vi "hidSPD Read Report (poly).vi"   [LabVIEW 2018, in "hidSPDLibForLabView.lvlib"]
uses:
  hidSPDLibForLabView.lvlib
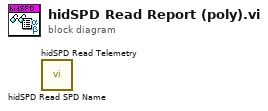
[diagram p0: block diagram]
diagram:
  n1 = call "hidSPD Read SPD Name.vi"() -> ()  [unwired: 9 in, 3 out]
  n2 = call "hidSPD Read Telemetry.vi"() -> ()  [unwired: 9 in, 3 out]
